vi "RX-SIM-BPCS-UDP (SubVI).vi"() -> (0 "BPCS-FJ":dbl, 1 "BPCS-10LI200":dbl, 2 "SIM-BPCS-RX-ARRAY":dbl[](array[numeric]), 3 "BPCS-10TI100":dbl)   [LabVIEW 2018]
panel:
  out "BPCS-10TI105":dbl
  out "BPCS-10AI300":dbl
  out "BPCS-F0":dbl
  out "BPCS-F":dbl
  out "BPCS-CA0":i16
  out "BPCS-TJ0":i16
  out "BPCS-T0":i16
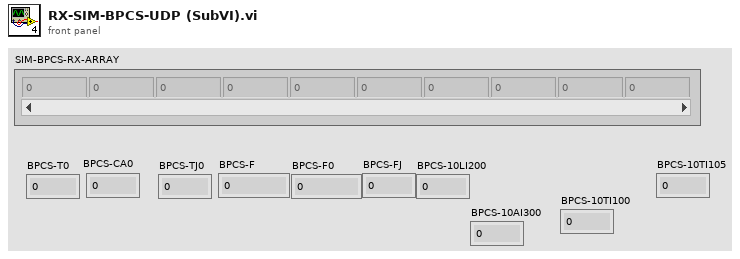
[diagram p1: front panel]
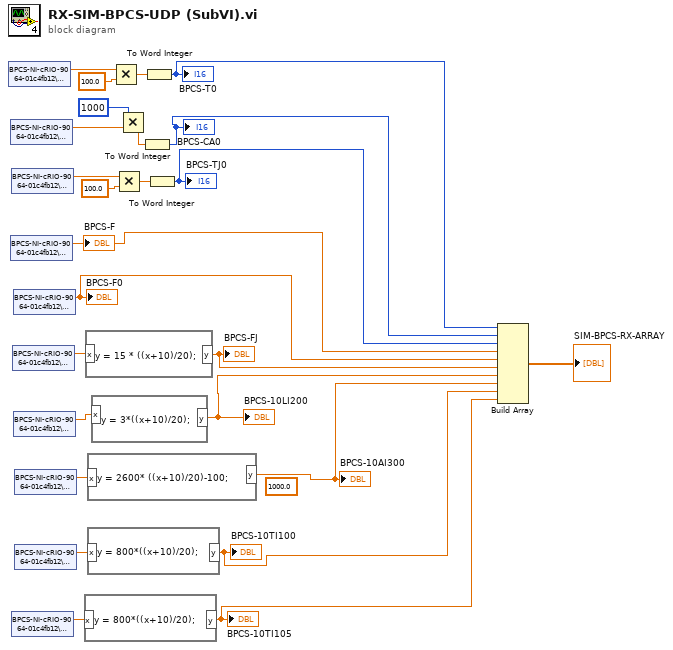
[diagram p0: block diagram]
diagram:
  (unwired) 1000.0 ("y")
  n1 = shared-variable "BPCS-NI-cRIO-9064-01c4fb12\\Mod2\\AI0"() -> (w25:dbl)  [unwired: 1 in, 1 out]
  n2 = shared-variable "BPCS-NI-cRIO-9064-01c4fb12\\Mod2\\AI1"() -> (w4:dbl)  [unwired: 1 in, 1 out]
  n3 = shared-variable "BPCS-NI-cRIO-9064-01c4fb12\\Mod2\\AI3"() -> (w13:dbl)  [unwired: 1 in, 1 out]
  "BPCS-F" <- w13
  n4 = shared-variable "BPCS-NI-cRIO-9064-01c4fb12\\Mod2\\AI2"() -> (w22:dbl)  [unwired: 1 in, 1 out]
  n5 = shared-variable "BPCS-NI-cRIO-9064-01c4fb12\\Mod2\\AI9"() -> (w16:dbl)  [unwired: 1 in, 1 out]
  n6 = shared-variable "BPCS-NI-cRIO-9064-01c4fb12\\Mod2\\AI5"() -> (w19:dbl)  [unwired: 1 in, 1 out]
  n7 = shared-variable "BPCS-NI-cRIO-9064-01c4fb12\\Mod2\\AI4"() -> (w12:dbl)  [unwired: 1 in, 1 out]
  "BPCS-F0" <- w12
  n8 = shared-variable "BPCS-NI-cRIO-9064-01c4fb12\\Mod2\\AI6"() -> (w7:dbl)  [unwired: 1 in, 1 out]
  n9 = shared-variable "BPCS-NI-cRIO-9064-01c4fb12\\Mod2\\AI7"() -> (w18:dbl)  [unwired: 1 in, 1 out]
  n10 = shared-variable "BPCS-NI-cRIO-9064-01c4fb12\\Mod2\\AI8"() -> (w17:dbl)  [unwired: 1 in, 1 out]
  n11 = formula code="y = 800*((x+10)/20);"("x"=w16) -> ("y"=w9:dbl)
  "BPCS-10TI105" <- w9
  n12 = formula code="y = 15 * ((x+10)/20);"("x"=w19) -> ("y"=w11:dbl)
  "BPCS-FJ" <- w11
  n13 = formula code="y = 2600* ((x+10)/20)-100;"("x"=w18) -> ("y"=w1:dbl)
  "BPCS-10AI300" <- w1
  n14 = formula code="y = 800*((x+10)/20);"("x"=w17) -> ("y"=w10:dbl)
  "BPCS-10TI100" <- w10
  n15 = formula code="y = 3*((x+10)/20);"("x"=w7) -> ("y"=w6:dbl)
  "BPCS-10LI200" <- w6
  n16 = Multiply(x=w25, y=100.0) -> (x*y=w23:dbl)
  n17 = Multiply(x=w22, y=100.0) -> (x*y=w20:dbl)
  n18 = Multiply(x=i16 1000, y=w4) -> (x*y=w3:dbl)
  n19 = To Word Integer(number=w3) -> (16bit integer=w2:i16)
  "BPCS-CA0" <- w2
  n20 = To Word Integer(number=w23) -> (16bit integer=w15:i16)
  "BPCS-T0" <- w15
  n21 = To Word Integer(number=w20) -> (16bit integer=w14:i16)
  "BPCS-TJ0" <- w14
  n22 = Build Array(w15, w2, w14, w13, w12, w11, w6, w1, w10, w9) -> (→"SIM-BPCS-RX-ARRAY":dbl[])
